vi "FB Overlay Global.vi"() -> ()   [LabVIEW 2017]
panel:
  in  "overlay refs":refnum<vi>[](array[refnum])
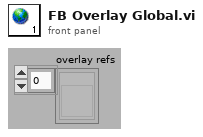
[diagram p1: front panel]
diagram:
